vi "dfd_Convert Integer Array to String.vi"(4 "append EOL?":bool=TRUE, 5 "indent order":i32, 6 "display in one line?":bool, 7 "width (-)":i16, 11 "I32 values":i32[](array[numeric])) -> (3 "string":string)   [LabVIEW 2017, in "NI_DigFilter_Process.lvlib"]
uses:
  <vilib>/addons/Digital Filter Design/NI_DigFilter_Process.lvlib
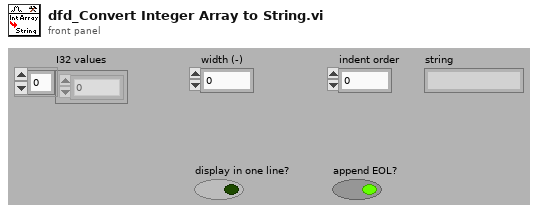
[diagram p1: front panel]
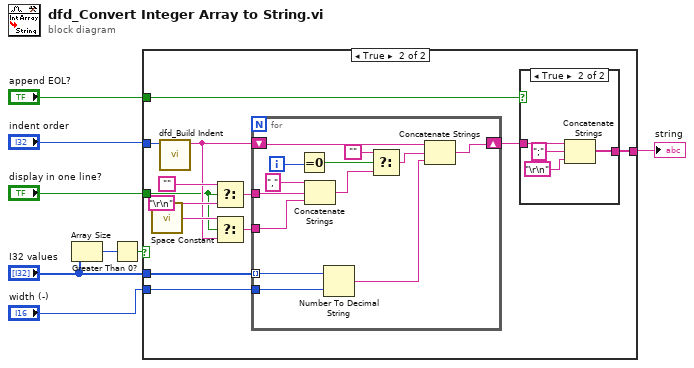
[diagram p0: block diagram]
diagram:
  n1 = Array Size(array="I32 values") -> (size(s)=w8:i32)
  n2 = Greater Than 0?(x=w8) -> (x > 0?=w4:bool)
  n3 = case shown="True" w4 {
    tunnel: "I32 values" -> [_ w21]
    tunnel: "indent order" -> [_ w18]
    tunnel: [_ w19] -> w7
    tunnel: "display in one line?" -> [_ w11]
    tunnel: "width (-)" -> [_ w10]
    tunnel: "append EOL?" -> [_ w9]
    frame False {
    }
    frame True {
      n4 = call <vilib>:"Space Constant.vi"() -> ("String"=w14:string)
      n5 = call <vilib>:"dfd_Build Indent.vi"("indent order"=w18) -> ("tag indent"=w12:string)  [unwired: 10 out]
      n6 = Select(t="", s=w11, f="\r\n") -> (s? t:f=w16:string)
      n7 = Select(t=w14, s=w11, f=w12) -> (s? t:f=w13:string)
      n8 = for {
        tunnel: w21 -> [w29] mode=indexing
        shift-right: [w38] -> w20
        shift-left: w12 -> [w37]
        tunnel: w16 -> [w34]
        tunnel: w13 -> [w31]
        tunnel: w10 -> [w27]
        i -> [w39]
        n9 = Equal To 0?(x=w39) -> (x = 0?=w32:bool)
        n10 = Concatenate Strings(",", w34, w31) -> (w33:string)
        n11 = Number To Decimal String(number=w29, width (-)=w27) -> (decimal integer string=w28:string)
        n12 = Select(t="", s=w32, f=w33) -> (s? t:f=w36:string)
        n13 = Concatenate Strings(w37, w36, w28) -> (w38:string)
      }
      n14 = case shown="True" w9 {
        tunnel: w20 -> [w22 w26]
        tunnel: [w22 w25] -> w19
        frame False {
        }
        frame True {
          n15 = Concatenate Strings(w26, ";" ("string"), "\r\n") -> (w25:string)
        }
      }
    }
  }
  "string" <- w7
